vi "frontPanel.vi"(8 "error in (no error)":errorcluster, 10 "ScriptEvent":refnum<class "ScriptEvent.lvclass">, 11 "ActionPanel in":refnum<class "ChangeValueAction.lvclass">) -> (0 "error out":errorcluster, 2 "ScriptEvent out":refnum<class "ScriptEvent.lvclass">, 3 "ActionPanel out":refnum<class "ChangeValueAction.lvclass">)   [LabVIEW 2011, in "Views.lvlib" / "ScriptEditor.lvlib" / "ChangeValueAction.lvclass"]
uses:
  ChangeValueAction.lvclass
  Tools/Scripting/ScriptingEvent/ScriptEvent.lvclass
  ChangeValueAction.lvclass/ChangeValueAction.ctl
  ActionPanel.lvclass
panel:
  out "editing":bool
  in  "States":u16(ring)
  out "ready?":bool
  in  "close":bool
  in  "Value":string
  in  "Dt":dbl format="%.6g"
  in  "Time":dbl format="%.6g"
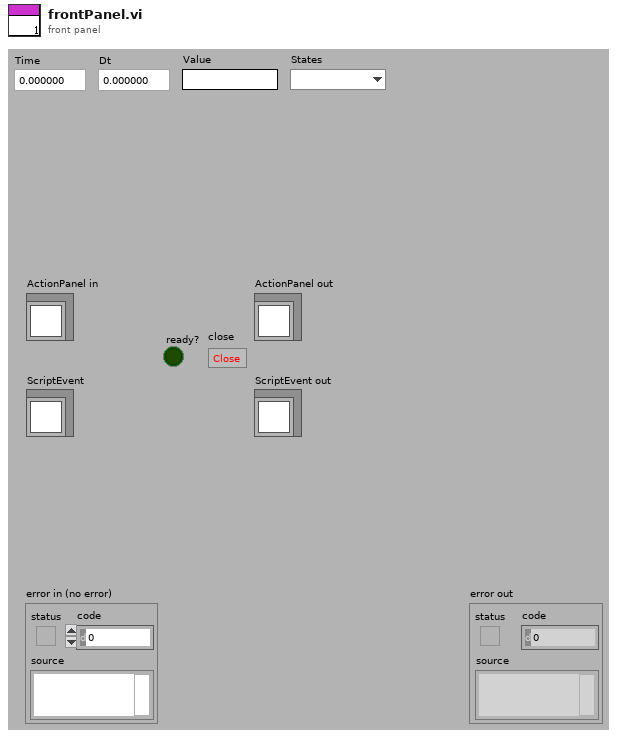
[diagram p1: front panel]
types:
  T1 = cluster{"Time":refnum<vi>, "Dt":refnum<vi>, "Value":refnum<vi>, "States":refnum<vi>}
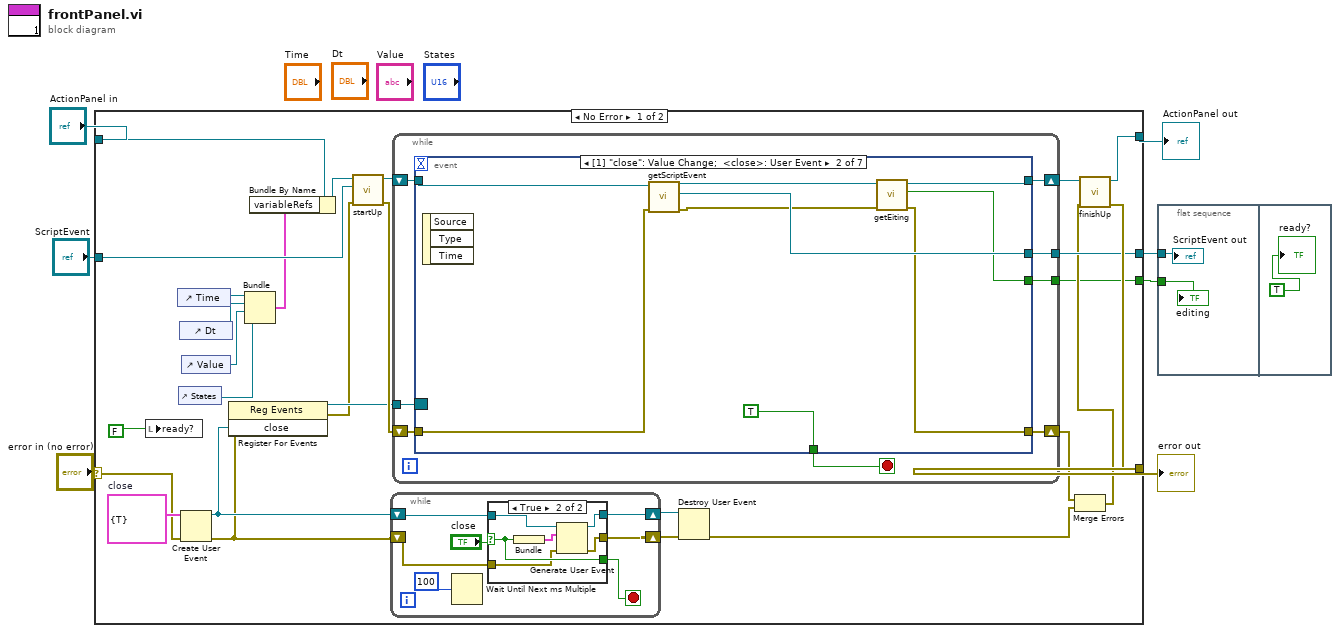
[diagram p0: block diagram]
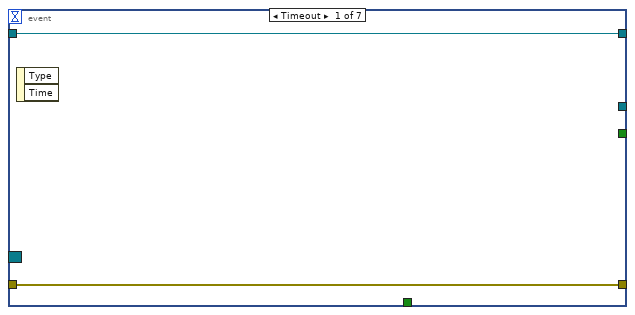
[diagram p3: hidden frame]
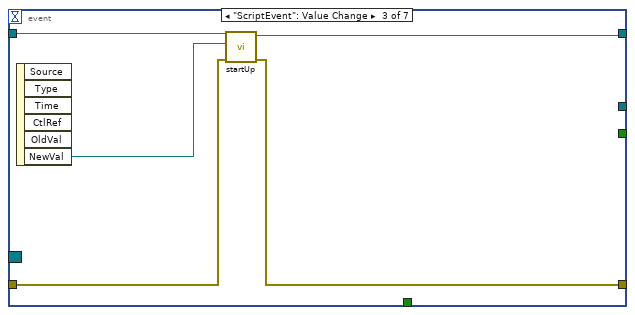
[diagram p4: hidden frame]
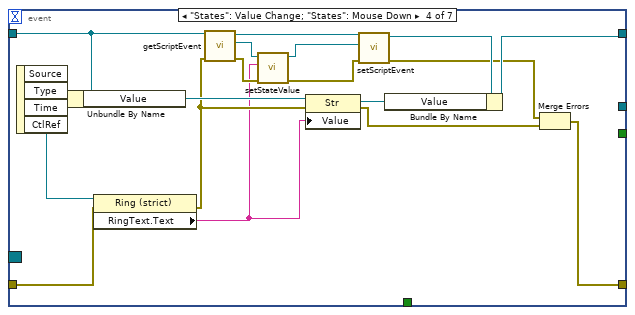
[diagram p5: hidden frame]
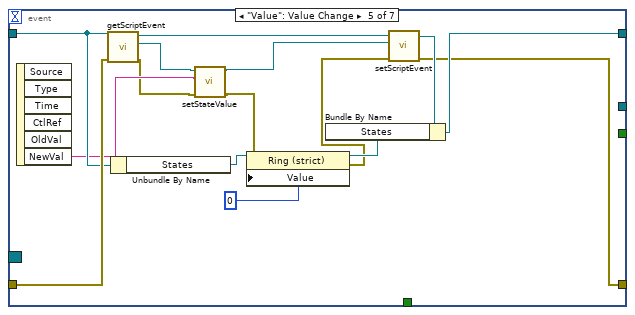
[diagram p6: hidden frame]
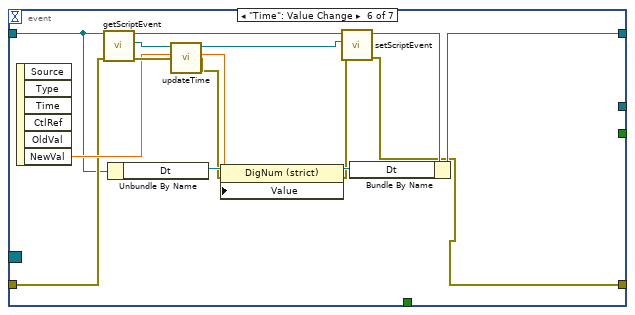
[diagram p7: hidden frame]
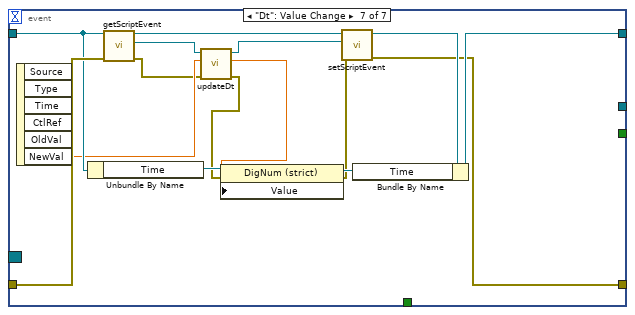
[diagram p8: hidden frame]
diagram:
  n1 = case shown="No Error" "error in (no error)" {
    selector: "error in (no error)" -> [w20 w137]
    tunnel: "ActionPanel in" -> [w10 w138]
    tunnel: [w26 w137] -> w5
    tunnel: [w27 w138] -> w3
    tunnel: "ScriptEvent" -> [w30 _]
    tunnel: [w24 _] -> w2
    tunnel: [w8 _] -> w1
    frame No Error {
      w21 = cluster{"close":bool} {"close"=TRUE}  # close
      n2 = local write "ready?"(FALSE) -> ()
      n3 = control-ref of="Time"() -> (w33:refnum<vi>)
      n4 = control-ref of="States"() -> (w23:refnum<vi>)
      n5 = control-ref of="Dt"() -> (w32:refnum<vi>)
      n6 = Create User Event(user event datatype=w21, error in=w20) -> (user event=w18:refnum<user-event>, error out=w15:errorcluster)
      n7 = control-ref of="Value"() -> (w31:refnum<vi>)
      n8 = register-events(error in=w15, w18) -> (reference out=w19:refnum<event-registration>, error out=w9:errorcluster)  [unwired: 1 in]
      n9 = Bundle("Time"=w33, "Dt"=w32, "Value"=w31, "States"=w23) -> (w22:T1)  [unwired: 1 in]
      n10 = Bundle By Name(cluster=w10, "variableRefs"=w22) -> (w11:refnum<class "ChangeValueAction.lvclass">)
      n11 = call-dynamic "startUp.vi"("error in (no error)"=w9, "ScriptEvent"=w30, "ChangeValueAction in"=w11) -> ("error out"=w29:errorcluster, "ChangeValueAction out"=w34:refnum<class "ChangeValueAction.lvclass">)  [unwired: 7 in]
      n12 = while {
        shift-right: [w37] -> w16
        shift-left: w15 -> [w36]
        shift-right: [w38] -> w17
        shift-left: w18 -> [w41]
        stop <- w39 stop-if-true
        n13 = Wait Until Next ms Multiple(millisecond multiple=100) -> ()  [unwired: 1 out]
        n14 = case shown="True" "close" {
          selector: "close" -> [w44 w48]
          tunnel: w41 -> [w43 w50]
          tunnel: [w44 w48] -> w39
          tunnel: [w43 w47] -> w38
          tunnel: [w42 w46] -> w37
          tunnel: w36 -> [w42 w45]
          frame False {
          }
          frame True {
            n15 = Bundle(w48) -> (w49:cluster{bool})  [unwired: 1 in]
            n16 = Generate User Event(user event=w50, event data cluster=w49, error in=w45) -> (user event out=w47:refnum<user-event>, error out=w46:errorcluster)
          }
        }
      }
      n17 = while {
        shift-right: [w58] -> w28
        shift-left: w34 -> [w57]
        shift-right: [w55] -> w14
        shift-left: w29 -> [w56]
        tunnel: [w53] -> w24
        tunnel: w19 -> [w52]
        tunnel: [w51] -> w8
        stop <- w54 stop-if-true
        n18 = event shown="[1] \"close\": Value Change;  <close>: User Event" {
          selector: w52 -> [_ _ _ _ _ _ _]
          dyn-events: _ -> [_ _ _ _ _ _ _]
          timeout: _ -> [_ _ _ _ _ _ _]
          tunnel: [w60 w64 w73 w80 w99 w110 w130] -> w58
          tunnel: w57 -> [w60 w69 w74 w86 w104 w116 w134]
          tunnel: [w59 w62 w70 w77 w97 w107 w128] -> w55
          tunnel: w56 -> [w59 w67 w71 w87 w105 w117 w135]
          tunnel: [_ TRUE _ _ _ _ _] -> w54
          tunnel: [_ w68 _ _ _ _ _] -> w53
          tunnel: [_ w61 _ _ _ _ _] -> w51
          event Timeout {
            n19 = event-data() -> ()  [unwired: 1 in, 2 out]
          }
          event "close": Value Change; User Event {
            n20 = event-data() -> ()  [unwired: 1 in, 3 out]
            n21 = call "getScriptEvent.vi"("error in (no error)"=w67, "ActionPanel.lvclass in"=w69) -> ("error out"=w63:errorcluster, "ScriptEvent.lvclass"=w68:refnum<class "ScriptEvent.lvclass">, "ActionPanel.lvclass out"=w65:refnum<class "ChangeValueAction.lvclass">)  [unwired: 7 in]
            n22 = call "getEiting.vi"("error in (no error)"=w63, "ActionPanel.lvclass in"=w65) -> ("error out"=w62:errorcluster, "editing?"=w61:bool, "ActionPanel.lvclass out"=w64:refnum<class "ChangeValueAction.lvclass">)  [unwired: 7 in]
          }
          event "ScriptEvent": Value Change {
            n23 = event-data() -> ("NewVal"=w72:refnum<class "ScriptEvent.lvclass">)  [unwired: 1 in, 5 out]
            n24 = call-dynamic "startUp.vi"("error in (no error)"=w71, "ScriptEvent"=w72, "ChangeValueAction in"=w74) -> ("error out"=w70:errorcluster, "ChangeValueAction out"=w73:refnum<class "ChangeValueAction.lvclass">)  [unwired: 7 in]
          }
          event "States": Value Change; "States": Mouse Down {
            n25 = event-data() -> ("CtlRef"=w88:refnum<vi>)  [unwired: 1 in, 3 out]
            n26 = Unbundle By Name(w86) -> ("Value"=w85:refnum<vi>)
            n27 = property class="Ring (strict)"(reference=w88, error in=w87) -> (error out=w84:errorcluster, "RingText.Text"=w83:string)  [unwired: 1 out]
            n28 = call "getScriptEvent.vi"("error in (no error)"=w84, "ActionPanel.lvclass in"=w86) -> ("error out"=w89:errorcluster, "ScriptEvent.lvclass"=w90:refnum<class "ScriptEvent.lvclass">, "ActionPanel.lvclass out"=w91:refnum<class "ChangeValueAction.lvclass">)  [unwired: 7 in]
            n29 = call "setStateValue.vi"("error in (no error)"=w89, "stateValue"=w83, "ScriptEvent in"=w90) -> ("error out"=w75:errorcluster, "ScriptEvent out"=w76:refnum<class "ScriptEvent.lvclass">)  [unwired: 7 in]
            n30 = property class="Str"(reference=w85, error in=w84, "Value"=w83) -> (reference out=w82:refnum<vi>, error out=w78:errorcluster)
            n31 = call "setScriptEvent.vi"("error in (no error)"=w75, "ScriptEvent.lvclass"=w76, "ActionPanel.lvclass in"=w91) -> ("error out"=w79:errorcluster, "ActionPanel.lvclass out"=w81:refnum<class "ChangeValueAction.lvclass">)  [unwired: 7 in]
            n32 = Bundle By Name(cluster=w81, "Value"=w82) -> (w80:refnum<class "ChangeValueAction.lvclass">)
            n33 = Merge Errors(w79, w78) -> (w77:errorcluster)
          }
          event "Value": Value Change {
            n34 = event-data() -> ("NewVal"=w94:string)  [unwired: 1 in, 5 out]
            n35 = call "getScriptEvent.vi"("error in (no error)"=w105, "ActionPanel.lvclass in"=w104) -> ("error out"=w93:errorcluster, "ScriptEvent.lvclass"=w96:refnum<class "ScriptEvent.lvclass">, "ActionPanel.lvclass out"=w106:refnum<class "ChangeValueAction.lvclass">)  [unwired: 7 in]
            n36 = Unbundle By Name(w104) -> ("States"=w103:refnum<vi>)
            n37 = call "setStateValue.vi"("error in (no error)"=w93, "stateValue"=w94, "ScriptEvent in"=w96) -> ("error out"=w92:errorcluster, "ScriptEvent out"=w95:refnum<class "ScriptEvent.lvclass">)  [unwired: 7 in]
            n38 = property class="Ring (strict)"(reference=w103, error in=w92, "Value"=0) -> (reference out=w100:refnum<vi>, error out=w98:errorcluster)
            n39 = call "setScriptEvent.vi"("error in (no error)"=w98, "ScriptEvent.lvclass"=w95, "ActionPanel.lvclass in"=w106) -> ("error out"=w97:errorcluster, "ActionPanel.lvclass out"=w101:refnum<class "ChangeValueAction.lvclass">)  [unwired: 7 in]
            n40 = Bundle By Name(cluster=w101, "States"=w100) -> (w99:refnum<class "ChangeValueAction.lvclass">)
          }
          event "Time": Value Change {
            n41 = event-data() -> ("NewVal"=w118:dbl)  [unwired: 1 in, 5 out]
            n42 = call "getScriptEvent.vi"("error in (no error)"=w117, "ActionPanel.lvclass in"=w116) -> ("error out"=w119:errorcluster, "ScriptEvent.lvclass"=w120:refnum<class "ScriptEvent.lvclass">, "ActionPanel.lvclass out"=w121:refnum<class "ChangeValueAction.lvclass">)  [unwired: 7 in]
            n43 = Unbundle By Name(w116) -> ("Dt"=w115:refnum<vi>)
            n44 = call "updateTime.vi"("error in (no error)"=w119, "time"=w118, "ScriptEvent in"=w120) -> ("error out"=w114:errorcluster, "dt"=w113:dbl, "ScriptEvent out"=w108:refnum<class "ScriptEvent.lvclass">)  [unwired: 6 in]
            n45 = property class="DigNum (strict)"(reference=w115, error in=w114, "Value"=w113) -> (reference out=w112:refnum<vi>, error out=w109:errorcluster)
            n46 = call "setScriptEvent.vi"("error in (no error)"=w109, "ScriptEvent.lvclass"=w108, "ActionPanel.lvclass in"=w121) -> ("error out"=w107:errorcluster, "ActionPanel.lvclass out"=w111:refnum<class "ChangeValueAction.lvclass">)  [unwired: 7 in]
            n47 = Bundle By Name(cluster=w111, "Dt"=w112) -> (w110:refnum<class "ChangeValueAction.lvclass">)
          }
          event "Dt": Value Change {
            n48 = event-data() -> ("NewVal"=w126:dbl)  [unwired: 1 in, 5 out]
            n49 = Unbundle By Name(w134) -> ("Time"=w133:refnum<vi>)
            n50 = call "getScriptEvent.vi"("error in (no error)"=w135, "ActionPanel.lvclass in"=w134) -> ("error out"=w125:errorcluster, "ScriptEvent.lvclass"=w127:refnum<class "ScriptEvent.lvclass">, "ActionPanel.lvclass out"=w136:refnum<class "ChangeValueAction.lvclass">)  [unwired: 7 in]
            n51 = call "updateDt.vi"("error in (no error)"=w125, "dt"=w126, "ScriptEvent in"=w127) -> ("error out"=w123:errorcluster, "time"=w124:dbl, "ScriptEvent out"=w122:refnum<class "ScriptEvent.lvclass">)  [unwired: 6 in]
            n52 = property class="DigNum (strict)"(reference=w133, error in=w123, "Value"=w124) -> (reference out=w132:refnum<vi>, error out=w129:errorcluster)
            n53 = call "setScriptEvent.vi"("error in (no error)"=w129, "ScriptEvent.lvclass"=w122, "ActionPanel.lvclass in"=w136) -> ("error out"=w128:errorcluster, "ActionPanel.lvclass out"=w131:refnum<class "ChangeValueAction.lvclass">)  [unwired: 7 in]
            n54 = Bundle By Name(cluster=w131, "Time"=w132) -> (w130:refnum<class "ChangeValueAction.lvclass">)
          }
        }
      }
      n55 = Destroy User Event(user event=w17, error in=w16) -> (error out=w12:errorcluster)
      n56 = Merge Errors(w14, w12) -> (w13:errorcluster)
      n57 = call-dynamic "finishUp.vi"("error in (no error)"=w13, "ChangeValueAction in"=w28) -> ("error out"=w26:errorcluster, "ChangeValueAction out"=w27:refnum<class "ChangeValueAction.lvclass">)  [unwired: 8 in]
    }
    frame Error {
    }
  }
  "error out" <- w5
  "ActionPanel out" <- w3
  n58 = flat-sequence {
    tunnel: w2 -> [w140]
    tunnel: w1 -> [w139]
    frame #0 {
      "ScriptEvent out" <- w140
      "editing" <- w139
    }
    frame #1 {
      "ready?" <- TRUE
    }
  }
